vi "tm_setarea.vi"(8 "error in (no error)":errorcluster, 10 "Sub Region":T1, 11 "Handle in":u32) -> (0 "error out":errorcluster, 3 "Handle out":u32)   [LabVIEW 2015]
uses:
  tmcamcon.dll
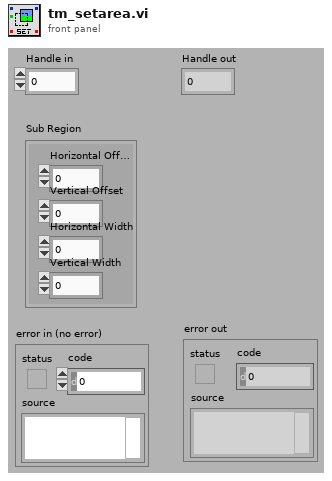
[diagram p1: front panel]
types:
  T1 = cluster{"Horizontal Offset":i32, "Vertical Offset":i32, "Horizontal Width":i32, "Vertical Width":i32}
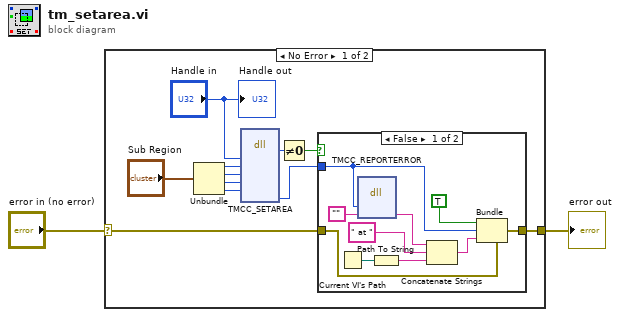
[diagram p0: block diagram]
diagram:
  n1 = case shown="No Error" "error in (no error)" {
    selector: "error in (no error)" -> [w4 w25]
    tunnel: [w3 w25] -> w1
    frame No Error {
      n2 = Unbundle("Sub Region") -> ("Horizontal Offset"=w8:i32, "Vertical Offset"=w9:i32, "Horizontal Width"=w10:i32, "Vertical Width"=w11:i32)
      n3 = dll-call lib="tmcamcon.dll" fn="TMCC_SETAREA"("HDCAM"="Handle in", "sho"=w8, "svo"=w9, "shw"=w10, "svw"=w11) -> ("return type"=w13:u32, "Erval"=w5:i32)  [unwired: 9 in, 2 out]
      n4 = Not Equal To 0?(x=w13) -> (x != 0?=w6:bool)
      n5 = case shown="False" w6 {
        tunnel: w4 -> [w23 w24]
        tunnel: [w22 w24] -> w3
        tunnel: w5 -> [w16 _]
        frame False {
          n6 = Current VI's Path() -> (path=w21:path)
          n7 = dll-call lib="tmcamcon.dll" fn="TMCC_REPORTERROR"("error"=w16, "buf"="") -> ("buf"=w15:string)  [unwired: 5 in, 2 out]
          n8 = Path To String(path=w21) -> (string=w17:string)
          n9 = Concatenate Strings(w15, " at ", w17) -> (w20:string)
          n10 = Bundle(cluster=w23, "status"=TRUE, "code"=w16, "source"=w20) -> (w22:errorcluster)
        }
        frame True {
        }
      }
      "Handle out" <- "Handle in"
    }
    frame Error {
    }
  }
  "error out" <- w1
